vi "GenerateXML.vi"(8 "error in (no error)":errorcluster, 11 "Preferences in":refnum<class "SetListPrefs.lvclass">) -> (0 "error out":errorcluster, 2 "FullXML":string, 3 "Preferences out":refnum<class "SetListPrefs.lvclass">)   [LabVIEW 2013, in "SetListPrefs.lvclass"]
uses:
  SetListPrefs.lvclass
  SetListPrefs.lvclass/SetListPrefs.ctl
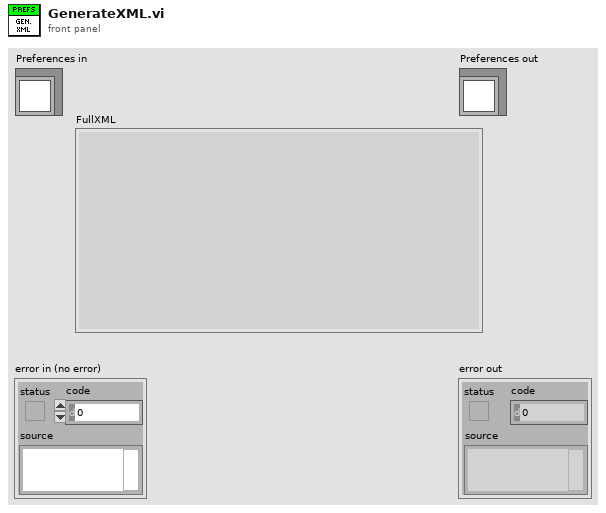
[diagram p1: front panel]
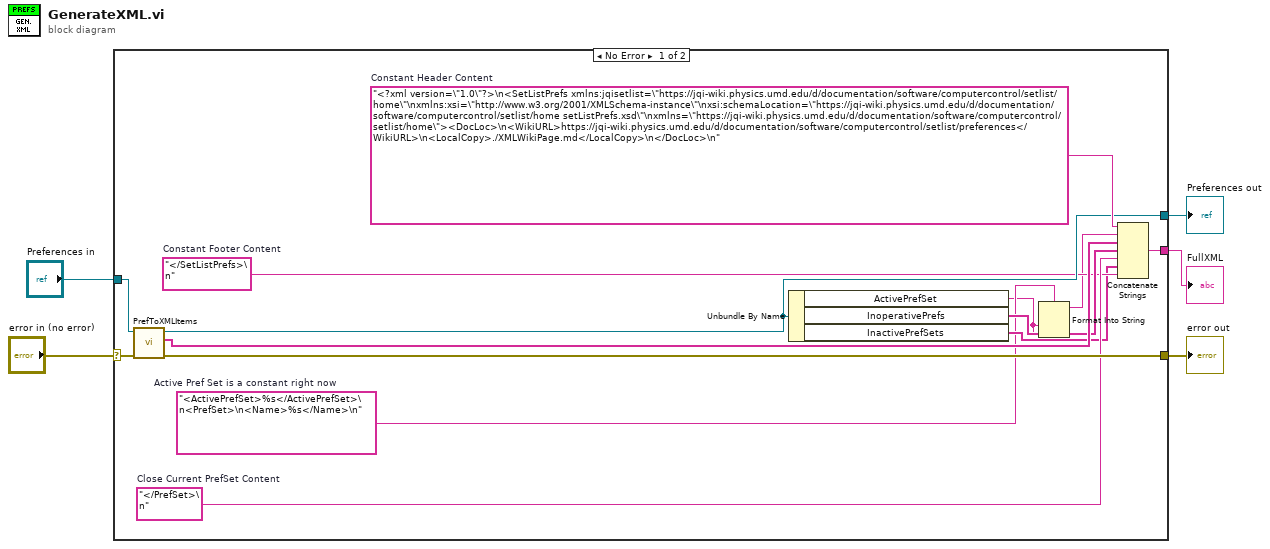
[diagram p0: block diagram]
diagram:
  n1 = case shown="No Error" "error in (no error)" {
    selector: "error in (no error)" -> [w16 w21]
    tunnel: [w15 w21] -> w4
    tunnel: [w13 w20] -> w2
    tunnel: "Preferences in" -> [w19 w20]
    tunnel: [w17 _] -> w1
    frame No Error {
      w11 = "</PrefSet>\n"  # Close Current PrefSet Content
      w10 = "</SetListPrefs>\n"  # Constant Footer Content
      w8 = "<ActivePrefSet>%s</ActivePrefSet>\n<PrefSet>\n<Name>%s</Name>\n"  # Active Pref Set is a constant right now
      w14 = "<?xml version=\"1.0\"?>\n<SetListPrefs xmlns:jqisetlist=\"https://jqi-wiki.physics.umd.edu/d/documentation/software/computercontrol/setlist/home\"\nxmlns:xsi=\"http://www.w3.org/2001/XMLSchema-instance\"\nxsi:schemaLocation=\"https://jqi-wiki.physics.umd.edu/d/documentation/software/computercontrol/setlist/home setListPrefs.xsd\"\nxmlns=\"https://jqi-wiki.physics.umd.edu/d/documentation/software/computercontrol/setlist/home\"><DocLoc>\n<WikiURL>https://jqi-wiki.physics.umd.edu/d/documentation/software/computercontrol/setlist/preferences</WikiURL>\n<LocalCopy>./XMLWikiPage.md</LocalCopy>\n</DocLoc>\n"  # Constant Header Content
      n2 = call "PrefToXMLItems.vi"("error in (no error)"=w16, "Preferences in"=w19) -> ("error out"=w15:errorcluster, "XMLArray"=w18:string[], "Preferences out"=w13:refnum<class "SetListPrefs.lvclass">)  [unwired: 7 in]
      n3 = Unbundle By Name(w13) -> ("ActivePrefSet"=w6:string, "InoperativePrefs"=w12:string[], "InactivePrefSets"=w9:string[])
      n4 = Format Into String(format string=w8, w6, w6) -> (resulting string=w7:string)  [unwired: 2 in, 1 out]
      n5 = Concatenate Strings(w14, w7, w18, w12, w11, w9, w10) -> (w17:string)
    }
    frame Error {
    }
  }
  "error out" <- w4
  "Preferences out" <- w2
  "FullXML" <- w1
